vi "4Pi Objective Image Alignment.vi"(7 "Calling VI Ref":refnum<vi>) -> ()   [LabVIEW 2016]
uses:
  4Pi OIA - Controls/4Pi OIA - ROI Selection.ctl
  4Pi OIA - Controls/4Pi OIA - Method.ctl
  4Pi OIA - Controls/4Pi OIA - Default Settings.ctl
  <vilib>/vision/Image Controls.llb/IMAQ Image.ctl
  4Pi OIA - Controls/4Pi OIA - Notifier Type.ctl
  4Pi OIA - Controls/4Pi OIA - Actions.ctl
  <vilib>/Utility/miscctls.llb/LVPointTypeDef.ctl
  Hardware Configuration/Hardware Configuration Controls/Device Function.ctl
  Hardware Configuration/Hardware Configuration Controls/Device Type.ctl
  Device Library/Cameras/Hamamatsu/Orca Flash/Orca Flash Controls/Orca Flash Actions.ctl
  Device Library/Shutters/Shutter Controls/Shutter Actions.ctl
  Device Library/Stages/Stages Controls/Stage Actions.ctl
  <resource>/objmgr/IMAQImage.rc
panel:
  in  "Main Tab":enum32{"Objective Alignment", "Settings"}(tab)
  in  "ROI Selection":T1
  in  "Image Selection":i32(ring) items=["Quad 01", "Quad 02", "Quad 03", "Quad 04"]
  in  "Method":T2
  in  "Align":bool
  in  "Frame Accumulations":u16=10
  in  "Alignment Cycles":u16=1
  out "Move Limit Error":bool
  in  "Save Default Config":bool
  in  "Objective Flip Ctrl":T3={"Flip X and Y"=FALSE, "Invert X"=FALSE, "Invert Y"=FALSE, "Camera Px. Size (µm)"=0.1, "Objective Move Limit (µm)"=1.0}
  in  "Get Shift":bool
  in  "Quit":bool
  # "For Debuggin Only"
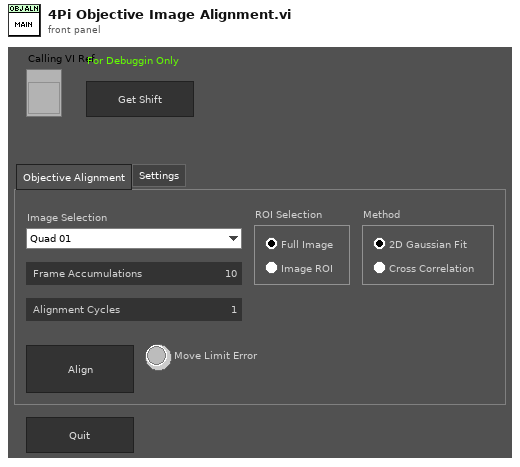
[diagram p1: front panel]
types:
  T1 = typedef "4Pi OIA - ROI Selection.ctl" = enum32{"Full Image", "ROI"}
  T2 = typedef "4Pi OIA - Method.ctl" = enum32{"2D Gaussian Fit", "Cross Correlation"}
  T3 = typedef "4Pi OIA - Default Settings.ctl" = cluster{"Flip X and Y":bool, "Invert X":bool, "Invert Y":bool, "Camera Px. Size (µm)":dbl, "Objective Move Limit (µm)":dbl}
  T4 = enum16{"Always On", "Always Off", "Off While Running"}
  T5 = typedef "LVPointTypeDef.ctl" = cluster{"Horizontal":i16, "Vertical":i16}
  T6 = typedef "4Pi OIA - Actions.ctl" = enum16{"Idle", "Start Alignment", "Get Upper Image", "Get Lower Image", "Get Shift", "Check Shift", "Move OBJ", "Quit"}
  T7 = enum8{"Enabled", "Disabled", "Disabled and Grayed Out"}
  T8 = typedef "4Pi OIA - Notifier Type.ctl" = cluster{"Action":T6, "ROI Selection":T1, "Method":T2, "Frame Accums.":u16, "Image Ref":T9, "OIA Default Settings":T3}
  T9 = typedef "IMAQ Image.ctl" = refnum<image>
  T10 = typedef "Device Function.ctl" = enum16{"Primary", "Secondary", "Overview", "Wide Field Drift Correction", "642 nm Excitation", "560 nm Excitation", "546 nm Excitation", "488 nm Excitation", "405 nm Excitation", "Objective Drift Correction", "Objective XY", "Objective Z", "Sample XY", "Sample Coarse Z", "Sample Z", "4Pi Lower", "4Pi Upper", "Adj Cavity", "Line Scanning", "Alert"}
  T11 = typedef "Device Type.ctl" = enum16{"AOTF", "Camera", "Deformable Mirror", "Laser", "Shutter", "Stage", "Waveform", "Email"}
  T12 = typedef "Orca Flash Actions.ctl" = enum16{"IDLE", "PREVIEW", "RECORD", "Record Settings", "SETPARAM", "GETPARAM", "SETROI", "GETROI", "PROGRESSIVE MODE", "AREA MODE", "STATUS", "QUIT"}
  T13 = typedef "Shutter Actions.ctl" = enum16{"Open", "Close", "Toggle", "Status", "Quit"}
  T14 = typedef "Stage Actions.ctl" = enum16{"Get Position", "MVR", "MOVE", "HALT", "ONTARGET", "ERROR", "REFERENCE", "INIT", "VELOCITY", "STATUS", "EXIT", "HOME", "ZEROPOS", "NANOPOS", "ANALOG", "QUIT"}
  T15 = enum32{"Invalid", "Standard", "Closed", "Hidden", "Minimized", "Maximized"}
  T16 = typedef "2D Gaussian - Best Fit Parameters.ctl" = cluster{"Amplitude":dbl, "X Position":dbl, "Y Position":dbl, "X Width":dbl, "Y Width":dbl, "Offset":dbl}
  T17 = typedef "LVRectTypeDef.ctl" = cluster{"Left":i16, "Top":i16, "Right":i16, "Bottom":i16}
  T18 = typedef "LVBoundsTypeDef.ctl" = cluster{"Width":u32, "Height":u32}
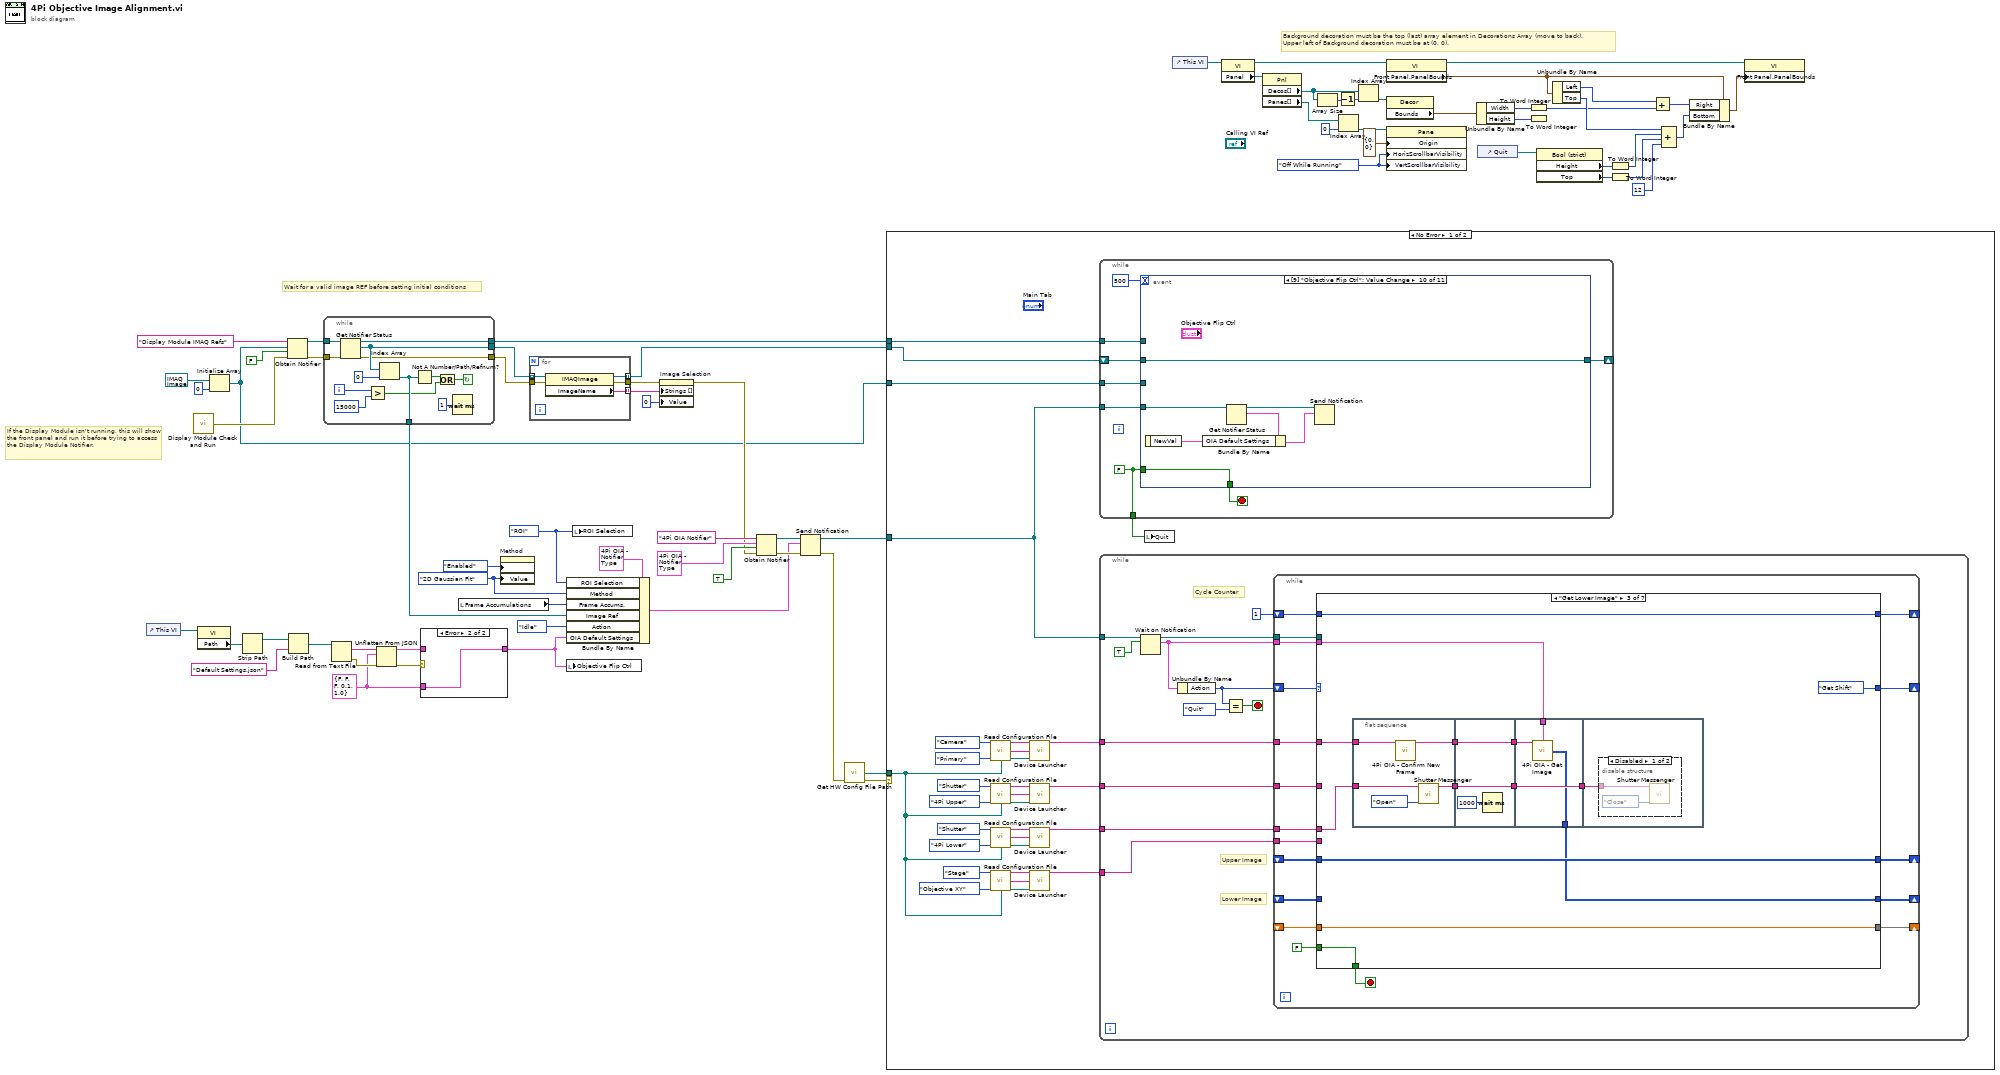
[diagram p0: block diagram]
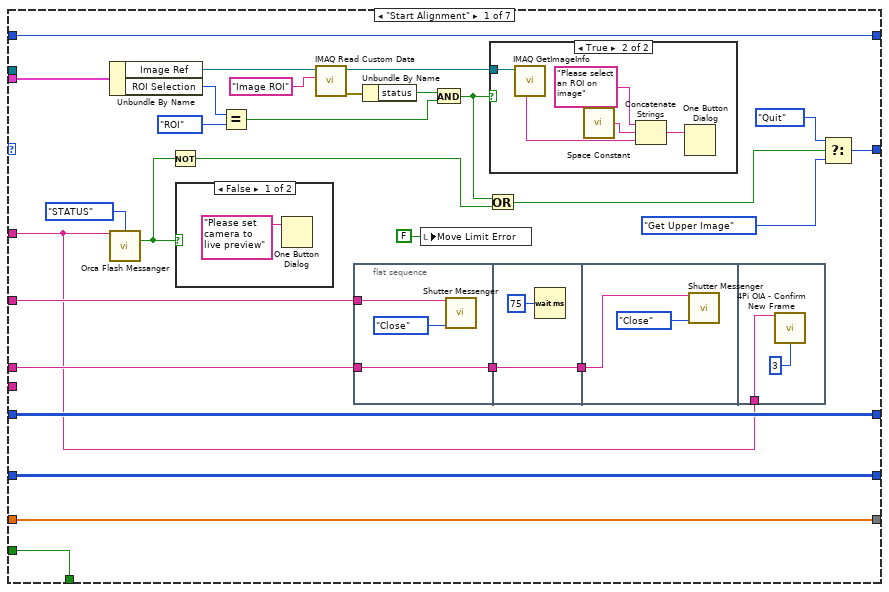
[diagram p3: hidden frame]
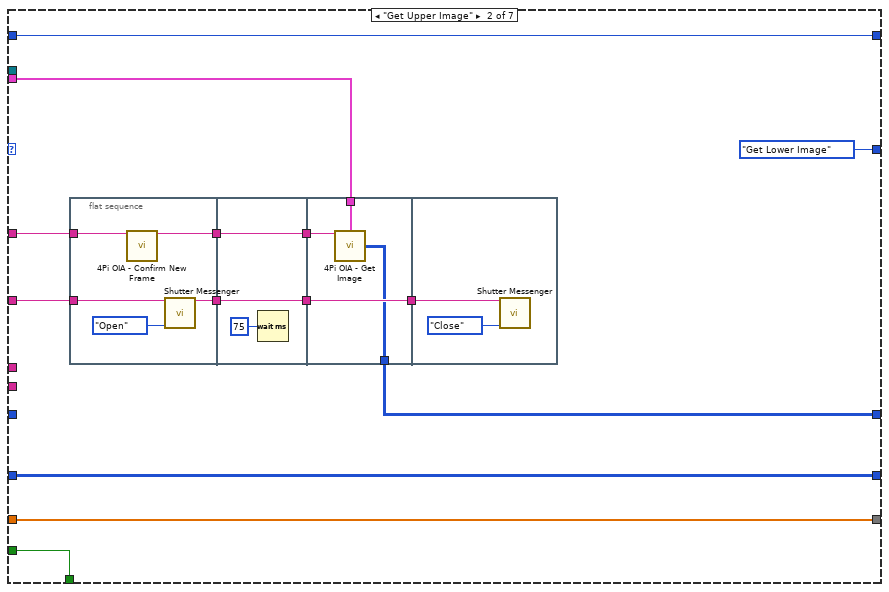
[diagram p6: hidden frame]
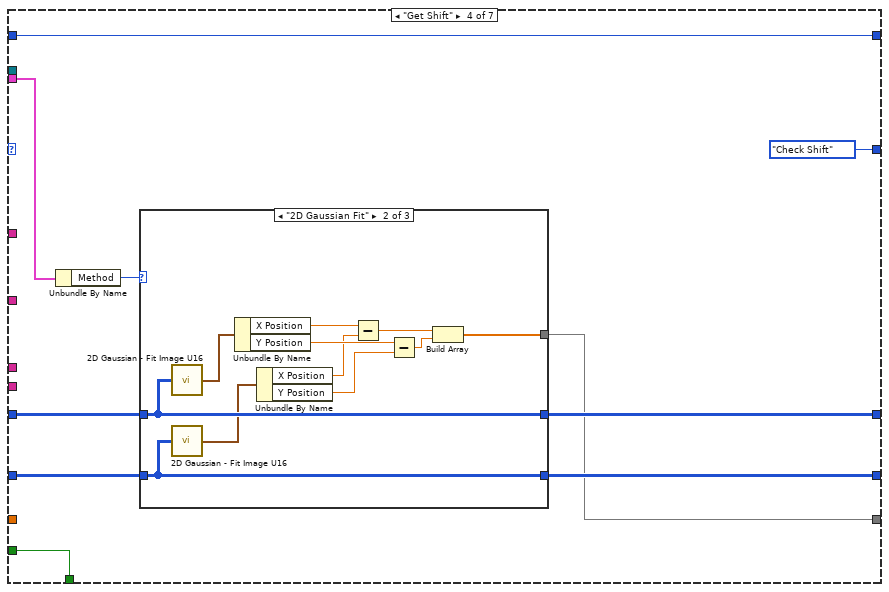
[diagram p8: hidden frame]
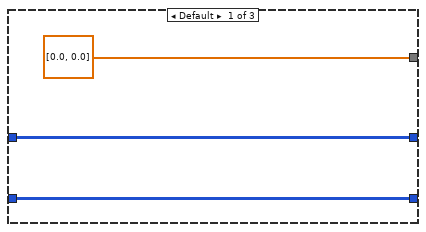
[diagram p9: hidden frame]
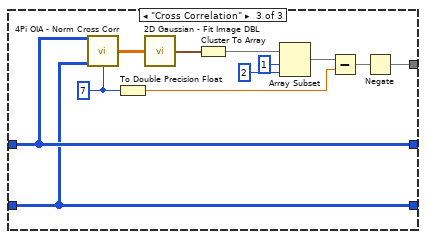
[diagram p10: hidden frame]
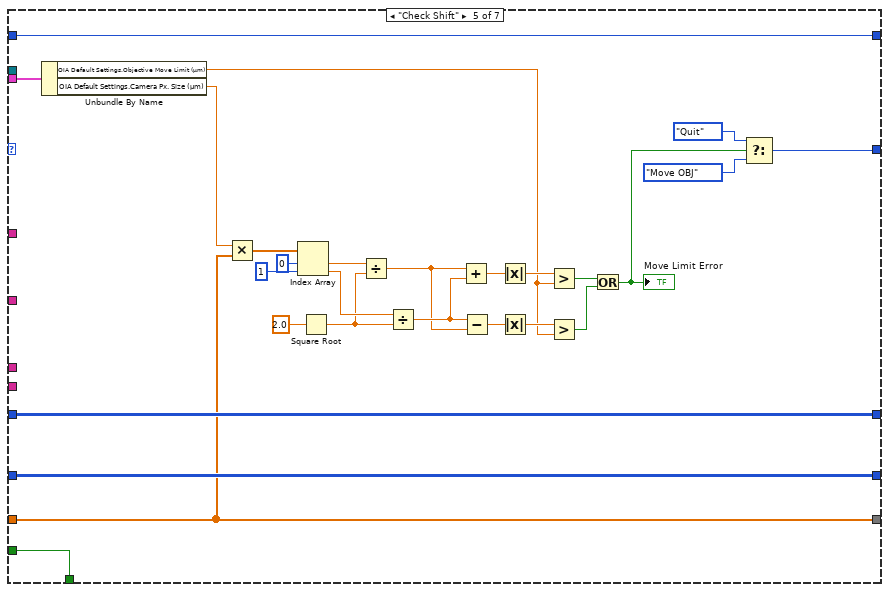
[diagram p11: hidden frame]
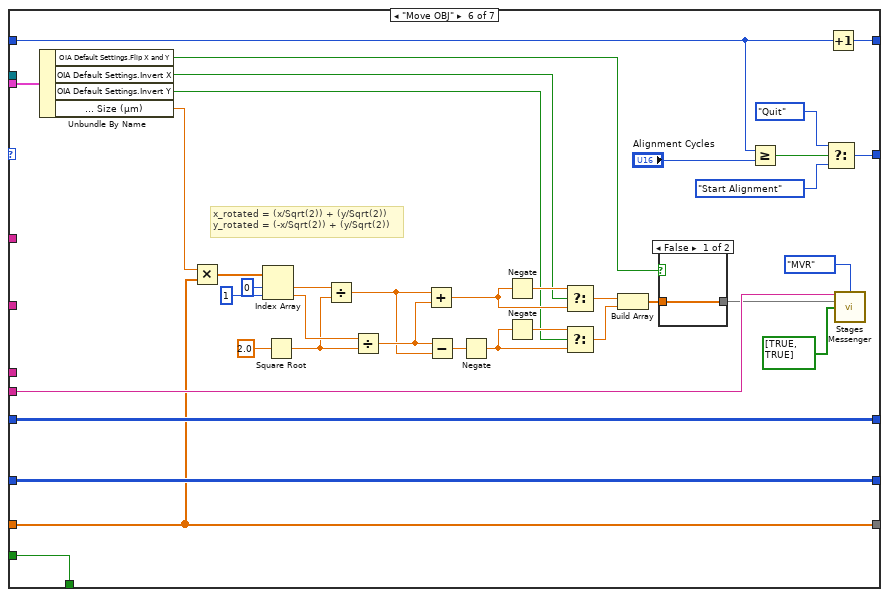
[diagram p12: hidden frame]
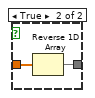
[diagram p13: hidden frame]
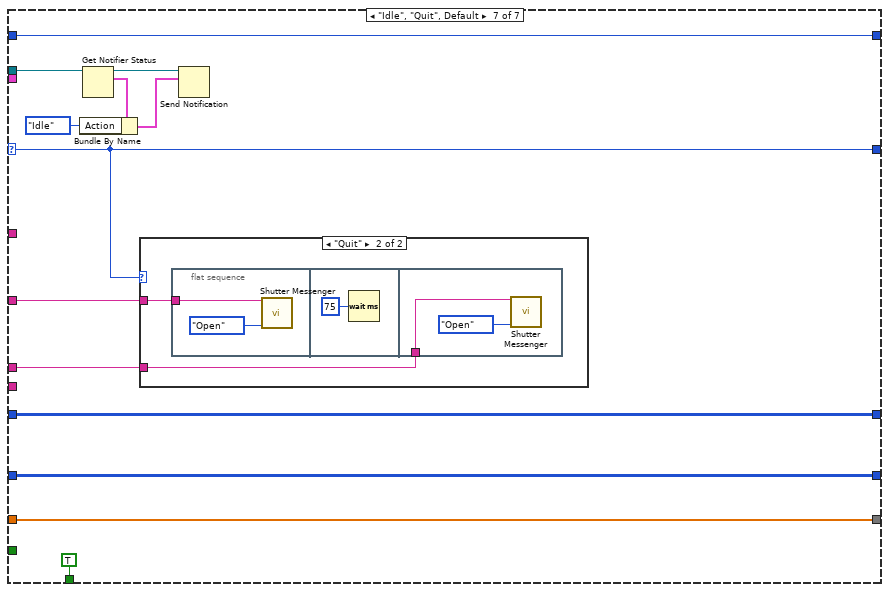
[diagram p14: hidden frame]
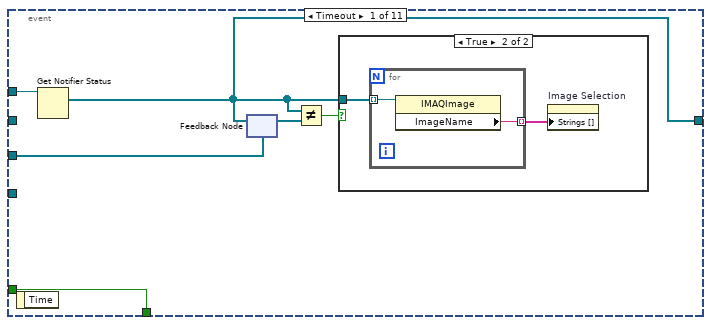
[diagram p16: hidden frame]
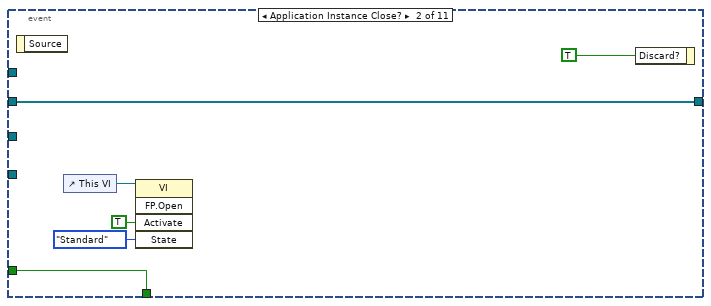
[diagram p18: hidden frame]
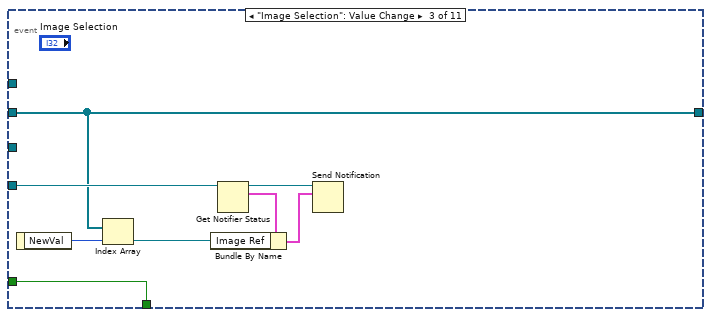
[diagram p19: hidden frame]
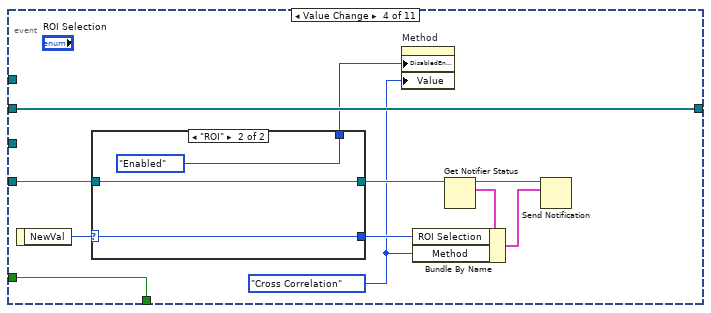
[diagram p20: hidden frame]
diagram:
  w2 = T3 {"Flip X and Y"=FALSE, "Invert X"=FALSE, "Invert Y"=FALSE, "Camera Px. Size (µm)"=0.1, "Objective Move Limit (µm)"=1.0} ("Objective Flip Type Def")
  w36 = T4."Off While Running" ("Vertical Scrollbar Visibility")
  w61 = 4Pi_OIA_-_Method."2D Gaussian Fit" ("Method")
  w62 = 4Pi_OIA_-_ROI_Selection."ROI" ("ROI Selection")
  # "Wait for a valid image REF before setting initial conditions"
  # "If the Display Module isn't running, this will show the front panel and run it before trying to access the Display Module Notifier."
  # "Background decoration must be the top (last) array element in Decorations Array (move to back).\nUpper left of Background decoration must be at (0, 0)."
  n1 = control-ref of="This VI"() -> (w8:refnum<vi>)
  n2 = call "Display Module Check and Run.vi"() -> ("Error"=w24:errorcluster)  [unwired: 15 in]
  n3 = property class="VI"(reference=w8) -> ("Path"=w9:path)  [unwired: 1 in, 2 out]
  n4 = Initialize Array(T9 refnum ("New Image"), 0 ("dimension size")) -> (w12:T9[])
  n5 = Strip Path(path=w9) -> (stripped path=w10:path)  [unwired: 1 out]
  n6 = Obtain Notifier(name (unnamed)="Display Module IMAQ Refs", notification data type=w12, create if not found? (T)=FALSE, error in (no error)=w24) -> (notifier out=w23:refnum<notifier>, error out=w22:errorcluster)  [unwired: 1 out]
  n7 = Build Path(base path=w10, name or relative path="Default Settings.json") -> (appended path=w7:path)
  n8 = while {
    tunnel: w23 -> [w86]
    tunnel: w22 -> [w85]
    tunnel: [w84] -> w21
    tunnel: [w83] -> w16
    tunnel: [w81] -> w20
    tunnel: [w79] -> w13
    i -> [w78]
    stop <- w75 continue-if-true
    n9 = Get Notifier Status(notifier=w86, error in (no error)=w85) -> (notifier out=w84:refnum<notifier>, current notification=w83:T9[], error out=w79:errorcluster)  [unwired: 2 out]
    n10 = Greater?(x=w78, y=15000) -> (0:w74:bool)
    n11 = Index Array(array=w83, index=0) -> (element=w81:T9)
    n12 = Not A Number/Path/Refnum?(number/path/refnum=w81) -> (NaN/Path/Refnum?=w76:bool)
    n13 = Or(x=w76, y=w74) -> (x .or. y?=w75:bool)
    n14 = Wait (ms)(milliseconds to wait=u32 1) -> ()  [unwired: 1 out]
  }
  n15 = Read from Text File(file (use dialog)=w7) -> (text=w6:string, error out=w5:errorcluster)  [unwired: 3 in, 2 out]
  n16 = Unflatten From JSON(JSON string=w6, type and defaults=w2, error in (no error)=w5) -> (value=w3:T3, error out=w4:errorcluster)  [unwired: 4 in]
  n17 = case shown="Error" w4 {
    tunnel: w3 -> [w87 _]
    tunnel: [w87 w88] -> w1
    tunnel: w2 -> [_ w88]
    frame No Error {
    }
    frame Error {
    }
  }
  n18 = local read "Frame Accumulations"() -> (w55:u16)
  n19 = property on="Method" class="RadioBtnsControl (strict)"("DisabledEnum"=T7."Enabled" ("Disabled"), "Value"=w61) -> ()  [unwired: 2 in, 2 out]
  n20 = for {
    tunnel: w16 -> [w93] mode=indexing
    tunnel: [w92] -> w19 mode=indexing
    tunnel: [w91] -> w17
    tunnel: [w90] -> w15 mode=indexing
    tunnel: w13 -> [w89]
    n21 = property class="IMAQImage"(reference=w93, error in=w89) -> (reference out=w90:T9, error out=w91:errorcluster, "ImageName"=w92:string)
  }
  n22 = Bundle By Name(cluster=T8 {"Action"=enum."Start Alignment", "ROI Selection"=enum."Full Image", "Method"=enum."2D Gaussian Fit", "Frame Accums."=0, "Image Ref"=refnum, "OIA Default Settings"={"Flip X and Y"=FALSE, "Invert X"=FALSE, "Invert Y"=FALSE, "Camera Px. Size (µm)"=0.1, "Objective Move Limit (µm)"=1.0}} ("4Pi OIA Notifier Type"), "ROI Selection"=w62, "Method"=w61, "Frame Accums."=w55, "Image Ref"=w20, "Action"=4Pi_OIA_-_Actions."Idle", "OIA Default Settings"=w1) -> (w57:T8)
  n23 = local write "Objective Flip Ctrl"(w1) -> ()
  n24 = local write "ROI Selection"(w62) -> ()
  n25 = property on="Image Selection" class="Ring (strict)"(error in=w17, "Strings []"=w19, "Value"=0) -> (error out=w14:errorcluster)  [unwired: 1 in, 1 out]
  n26 = Obtain Notifier(name (unnamed)="4Pi OIA Notifier", notification data type=T8 {"Action"=enum."Start Alignment", "ROI Selection"=enum."Full Image", "Method"=enum."2D Gaussian Fit", "Frame Accums."=0, "Image Ref"=refnum, "OIA Default Settings"={"Flip X and Y"=FALSE, "Invert X"=FALSE, "Invert Y"=FALSE, "Camera Px. Size (µm)"=0.1, "Objective Move Limit (µm)"=1.0}} ("4Pi OIA Notifier Type"), create if not found? (T)=TRUE, error in (no error)=w14) -> (notifier out=w60:refnum<notifier>, error out=w58:errorcluster)  [unwired: 1 out]
  n27 = Send Notification(notification=w57, notifier=w60, error in (no error)=w58) -> (notifier out=w59:refnum<notifier>, error out=w56:errorcluster)
  n28 = call "Get HW Config File Path.vi"("Error"=w56) -> ("File Path"=w72:path, "Error"=w73:errorcluster)  [unwired: 13 in]
  n29 = case shown="No Error" w73 {
    tunnel: w72 -> [w122 _]
    tunnel: w21 -> [w121 _]
    tunnel: w12 -> [w120 _]
    tunnel: w59 -> [w118 _]
    tunnel: w15 -> [w119 _]
    frame No Error {
      n30 = call "Read Configuration File.vi"("Device Type"=Device_Type."Camera", "Device Function"=Device_Function."Primary", "Config File Path"=w122) -> ("Unique Notifier Name"=w112:string, "Device Ports/IDs/Channels"=w114:string[], "Device Engine Path"=w113:path)  [unwired: 9 in, 1 out]
      n31 = call "Read Configuration File.vi"("Device Type"=Device_Type."Shutter", "Device Function"=Device_Function."4Pi Upper", "Config File Path"=w122) -> ("Unique Notifier Name"=w97:string, "Device Ports/IDs/Channels"=w99:string[], "Device Engine Path"=w98:path)  [unwired: 9 in, 1 out]
      n32 = call "Read Configuration File.vi"("Device Type"=Device_Type."Shutter", "Device Function"=Device_Function."4Pi Lower", "Config File Path"=w122) -> ("Unique Notifier Name"=w102:string, "Device Ports/IDs/Channels"=w100:string[], "Device Engine Path"=w101:path)  [unwired: 9 in, 1 out]
      n33 = call "Read Configuration File.vi"("Device Type"=Device_Type."Stage", "Device Function"=Device_Function."Objective XY", "Config File Path"=w122) -> ("Unique Notifier Name"=w107:string, "Device Ports/IDs/Channels"=w109:string[], "Device Engine Path"=w108:path)  [unwired: 9 in, 1 out]
      n34 = call "Device Launcher.vi"("Notifier Name"=w112, "Device Ports/IDs/Channels"=w114, "Device Engine Path"=w113) -> ("Notifier Name"=w117:string)  [unwired: 11 in, 1 out]
      n35 = call "Device Launcher.vi"("Notifier Name"=w97, "Device Ports/IDs/Channels"=w99, "Device Engine Path"=w98) -> ("Notifier Name"=w116:string)  [unwired: 11 in, 1 out]
      n36 = call "Device Launcher.vi"("Notifier Name"=w102, "Device Ports/IDs/Channels"=w100, "Device Engine Path"=w101) -> ("Notifier Name"=w115:string)  [unwired: 11 in, 1 out]
      n37 = call "Device Launcher.vi"("Notifier Name"=w107, "Device Ports/IDs/Channels"=w109, "Device Engine Path"=w108) -> ("Notifier Name"=w94:string)  [unwired: 11 in, 1 out]
      n38 = while {
        tunnel: [w382] -> w123
        tunnel: w121 -> [w381]
        tunnel: w120 -> [w380]
        tunnel: w118 -> [w379]
        shift-right: [w378] -> _
        shift-left: w119 -> [w377]
        stop <- w383 stop-if-true
        w382 = FALSE
        n39 = event shown="[9] \"Objective Flip Ctrl\": Value Change" {
          selector: _ -> [_ _ _ _ _ _ _ _ _ _ _]
          dyn-events: _ -> [_ _ _ _ _ _ _ _ _ _ _]
          timeout: 500 -> [_ _ _ _ _ _ _ _ _ _ _]
          tunnel: w382 -> [w390 w399 w408 w418 w432 w439 w446 w453 w463 w471 _]
          tunnel: [w390 w399 w408 w418 w432 w439 w446 w453 w463 w471 w478] -> w383
          tunnel: w381 -> [w389 _ _ _ _ _ _ _ _ _ _]
          tunnel: w380 -> [w388 _ _ _ _ _ _ _ _ _ _]
          tunnel: w379 -> [_ _ w407 w413 w427 w434 w445 w452 w462 w468 w472]
          tunnel: [w387 w395 w401 w419 w431 w438 w440 w447 w464 w469 w477] -> w378
          tunnel: w377 -> [_ w395 w401 w419 w431 w438 w440 w447 w464 w469 w477]
          event Timeout {
            n40 = event-data() -> ()  [unwired: 1 in, 1 out]
            n41 = Get Notifier Status(notifier=w389) -> (current notification=w387:T9[])  [unwired: 1 in, 4 out]
            n42 = feedback #1(w388) -> (w386:T9[])
            n43 = feedback-in #1(w387) -> ()
            n44 = Not Equal?(x=w387, y=w386) -> (x != y?=w385:bool)
            n45 = case shown="True" w385 {
              tunnel: w387 -> [_ w392]
              frame False {
              }
              frame True {
                n46 = for {
                  tunnel: w392 -> [w394] mode=indexing
                  tunnel: [w393] -> w391 mode=indexing
                  n47 = property class="IMAQImage"(reference=w394) -> ("ImageName"=w393:string)  [unwired: 1 in, 2 out]
                }
                n48 = property on="Image Selection" class="Ring (strict)"("Strings []"=w391) -> ()  [unwired: 2 in, 2 out]
              }
            }
          }
          event Application Instance Close? {
            n49 = event-data() -> ()  [unwired: 1 in, 1 out]
            n50 = control-ref of="This VI"() -> (w396:refnum<vi>)
            n51 = invoke class="VI" method="FP.Open"(reference=w396, "Activate"=TRUE ("Activate?"), "State"=T15."Standard") -> ()  [unwired: 2 in, 5 out]
            n52 = event-data("Discard?"=TRUE) -> ()  [unwired: 1 in, 1 out]
          }
          event "Image Selection": Value Change {
            n53 = event-data() -> ("NewVal"=w403:i32)  [unwired: 1 in]
            n54 = Index Array(array=w401, index=w403) -> (element=w402:T9)
            n55 = Get Notifier Status(notifier=w407) -> (notifier out=w406:refnum<notifier>, current notification=w405:T8)  [unwired: 1 in, 3 out]
            n56 = Bundle By Name(cluster=w405, "Image Ref"=w402) -> (w404:T8)
            n57 = Send Notification(notification=w404, notifier=w406) -> ()  [unwired: 1 in, 2 out]
          }
          event Value Change {
            w409 = 4Pi_OIA_-_Method."Cross Correlation" ("Method")
            n58 = event-data() -> ("NewVal"=w414:T1)  [unwired: 1 in]
            n59 = case shown="\"ROI\"" w414 {
              selector: w414 -> [w422 w424]
              tunnel: w413 -> [w421 w425]
              tunnel: [w422 w424] -> w411
              tunnel: [w421 w425] -> w412
              tunnel: [T7."Disabled and Grayed Out" ("Disabled") T7."Enabled" ("Disabled")] -> w410
              frame "Full Image", Default {
              }
              frame "ROI" {
              }
            }
            n60 = property on="Method" class="RadioBtnsControl (strict)"("DisabledEnum"=w410, "Value"=w409) -> ()  [unwired: 2 in, 2 out]
            n61 = Get Notifier Status(notifier=w412) -> (notifier out=w417:refnum<notifier>, current notification=w416:T8)  [unwired: 1 in, 3 out]
            n62 = Bundle By Name(cluster=w416, "ROI Selection"=w411, "Method"=w409) -> (w415:T8)
            n63 = Send Notification(notification=w415, notifier=w417) -> ()  [unwired: 1 in, 2 out]
          }
          event Value Change {
            n64 = event-data() -> ("NewVal"=w426:T2)  [unwired: 1 in]
            n65 = Get Notifier Status(notifier=w427) -> (notifier out=w430:refnum<notifier>, current notification=w429:T8)  [unwired: 1 in, 3 out]
            n66 = Bundle By Name(cluster=w429, "Method"=w426) -> (w428:T8)
            n67 = Send Notification(notification=w428, notifier=w430) -> ()  [unwired: 1 in, 2 out]
          }
          event "Frame Accumulations": Value Change {
            n68 = event-data() -> ("NewVal"=w433:u16)  [unwired: 1 in]
            n69 = Get Notifier Status(notifier=w434) -> (notifier out=w437:refnum<notifier>, current notification=w436:T8)  [unwired: 1 in, 3 out]
            n70 = Bundle By Name(cluster=w436, "Frame Accums."=w433) -> (w435:T8)
            n71 = Send Notification(notification=w435, notifier=w437) -> ()  [unwired: 1 in, 2 out]
          }
          event "Align": Value Change {
            n72 = event-data() -> ()  [unwired: 1 in, 1 out]
            n73 = Get Notifier Status(notifier=w445) -> (notifier out=w444:refnum<notifier>, current notification=w443:T8)  [unwired: 1 in, 3 out]
            n74 = Bundle By Name(cluster=w443, "Action"=4Pi_OIA_-_Actions."Start Alignment") -> (w442:T8)
            n75 = Send Notification(notification=w442, notifier=w444) -> ()  [unwired: 1 in, 2 out]
          }
          event "Get Shift": Value Change {
            # "For debugging only"
            n76 = event-data() -> ()  [unwired: 1 in, 1 out]
            n77 = Get Notifier Status(notifier=w452) -> (notifier out=w451:refnum<notifier>, current notification=w450:T8)  [unwired: 1 in, 3 out]
            n78 = Bundle By Name(cluster=w450, "Action"=4Pi_OIA_-_Actions."Get Shift") -> (w449:T8)
            n79 = Send Notification(notification=w449, notifier=w451) -> ()  [unwired: 1 in, 2 out]
          }
          event "Save Default Config": Value Change {
            n80 = event-data() -> ()  [unwired: 1 in, 1 out]
            n81 = Get Notifier Status(notifier=w462) -> (current notification=w456:T8)  [unwired: 1 in, 4 out]
            n82 = control-ref of="This VI"() -> (w461:refnum<vi>)
            n83 = Unbundle By Name(w456) -> ("OIA Default Settings"=w455:T3)
            n84 = property class="VI"(reference=w461) -> ("Path"=w460:path)  [unwired: 1 in, 2 out]
            n85 = Strip Path(path=w460) -> (stripped path=w459:path)  [unwired: 1 out]
            n86 = Flatten To JSON(anything=w455) -> (JSON string=w454:string)  [unwired: 2 in, 1 out]
            n87 = Build Path(base path=w459, name or relative path="Default Settings.json") -> (appended path=w457:path)
            n88 = Write to Text File(file (use dialog)=w457, text=w454) -> ()  [unwired: 2 in, 3 out]
          }
          event Value Change {
            n89 = event-data() -> ("NewVal"=w466:T3)  [unwired: 1 in]
            n90 = Get Notifier Status(notifier=w468) -> (notifier out=w470:refnum<notifier>, current notification=w467:T8)  [unwired: 1 in, 3 out]
            n91 = Bundle By Name(cluster=w467, "OIA Default Settings"=w466) -> (w465:T8)
            n92 = Send Notification(notification=w465, notifier=w470) -> ()  [unwired: 1 in, 2 out]
          }
          event "Quit": Value Change {
            n93 = event-data() -> ("NewVal"=w478:bool)  [unwired: 1 in]
            n94 = Get Notifier Status(notifier=w472) -> (notifier out=w473:refnum<notifier>, current notification=w474:T8)  [unwired: 1 in, 3 out]
            n95 = Bundle By Name(cluster=w474, "Action"=4Pi_OIA_-_Actions."Quit") -> (w475:T8)
            n96 = Send Notification(notification=w475, notifier=w473) -> ()  [unwired: 1 in, 2 out]
          }
        }
      }
      n97 = while {
        tunnel: w118 -> [w135]
        tunnel: w117 -> [w130]
        tunnel: w116 -> [w129]
        tunnel: w115 -> [w128]
        tunnel: w94 -> [w125]
        stop <- w132 stop-if-true
        # "Cycle Counter"
        # "Lower Image"
        # "Upper Image"
        n98 = Wait on Notification(notifier=w135, ignore previous (F)=TRUE) -> (notifier out=w126:refnum<notifier>, notification=w127:T8)  [unwired: 2 in, 2 out]
        n99 = Unbundle By Name(w127) -> ("Action"=w131:T6)
        n100 = Equal?(x=w131, y=4Pi_OIA_-_Actions."Quit") -> (x = y?=w132:bool)
        n101 = while {
          shift-right: [w150] -> _
          shift-left: w131 -> [w153]
          tunnel: w130 -> [w149]
          tunnel: w129 -> [w148]
          tunnel: w128 -> [w147]
          shift-right: [w144] -> _
          shift-left: _ -> [w143]
          shift-right: [w146] -> _
          shift-left: _ -> [w145]
          tunnel: w127 -> [w142]
          tunnel: w126 -> [w141]
          tunnel: w125 -> [w140]
          shift-right: [w139] -> _
          shift-left: _ -> [w138]
          shift-right: [w136] -> _
          shift-left: u16 1 -> [w137]
          stop <- w151 stop-if-true
          n102 = case shown="\"Get Lower Image\"" w153 {
            selector: w153 -> [_ _ _ _ _ _ w359]
            tunnel: FALSE -> [w181 w209 w237 w262 w315 w353 _]
            tunnel: [w181 w209 w237 w262 w315 w353 TRUE] -> w151
            tunnel: [w166 4Pi_OIA_-_Actions."Get Lower Image" ("Action") 4Pi_OIA_-_Actions."Get Shift" ("Action") 4Pi_OIA_-_Actions."Check Shift" ("Action") w291 w332 w359] -> w150
            tunnel: w149 -> [w158 w200 w231 _ _ _ _]
            tunnel: w148 -> [w164 w208 _ _ _ _ w358]
            tunnel: w147 -> [w163 _ w228 _ _ _ w357]
            tunnel: [w160 w202 w229 w256 w313 w351 w367] -> w146
            tunnel: w145 -> [w160 w202 _ w258 w313 w351 w367]
            tunnel: [w159 w201 w230 w257 w314 w352 w368] -> w144
            tunnel: w143 -> [w159 _ w230 w259 w314 w352 w368]
            tunnel: w142 -> [w157 w199 w227 w260 w302 w329 _]
            tunnel: w141 -> [_ _ _ _ _ _ w362]
            tunnel: w140 -> [_ _ _ _ _ w350 _]
            tunnel: [w156 w198 w226 w255 w303 w338 w361] -> w139
            tunnel: w138 -> [w156 w198 w226 _ w303 w338 w361]
            tunnel: w137 -> [w155 w197 w225 w254 w316 w331 w360]
            tunnel: [w155 w197 w225 w254 w316 w330 w360] -> w136
            frame "Start Alignment" {
              n103 = Unbundle By Name(w157) -> ("Image Ref"=w178:T9, "ROI Selection"=w180:T1)
              n104 = call "Orca Flash Messanger.vi"("Notifier Name"=w158, "Camera Actions"=Orca_Flash_Actions."STATUS") -> ("Running?"=w170:bool)  [unwired: 9 in, 4 out]
              n105 = Not(x=w170) -> (.not. x?=w169:bool)
              n106 = case shown="False" w170 {
                frame False {
                  n107 = One Button Dialog(message="Please set camera to live preview") -> ()  [unwired: 1 in, 1 out]
                }
                frame True {
                }
              }
              n108 = Equal?(x=w180, y=4Pi_OIA_-_ROI_Selection."ROI") -> (x = y?=w174:bool)
              n109 = call "IMAQ Read Custom Data"("Key"="Image ROI", "Image"=w178) -> ("error out"=w176:errorcluster, "Image (duplicate)"=w173:T9)  [unwired: 7 in, 1 out]
              n110 = flat-sequence {
                tunnel: w164 -> [w183]
                tunnel: w163 -> [w182]
                tunnel: [w182] -> w162
                tunnel: w162 -> [w186]
                tunnel: [w186] -> w161
                tunnel: w161 -> [w187]
                tunnel: w158 -> [w190]
                frame #0 {
                  n111 = call "Shutter Messenger.vi"("Notifier Name"=w183, "Action"=Shutter_Actions."Close") -> ()  [unwired: 12 in, 2 out]
                }
                frame #1 {
                  n112 = Wait (ms)(milliseconds to wait=u32 75) -> ()  [unwired: 1 out]
                }
                frame #2 {
                  n113 = call "Shutter Messenger.vi"("Notifier Name"=w187, "Action"=Shutter_Actions."Close") -> ()  [unwired: 12 in, 2 out]
                }
                frame #3 {
                  n114 = call "4Pi OIA - Confirm New Frame.vi"("Camera Notifier Name"=w190, "Wait No. (1)"=u32 3 ("Wait No.")) -> ()  [unwired: 13 in, 1 out]
                }
              }
              n115 = Unbundle By Name(w176) -> ("status"=w175:bool)
              n116 = local write "Move Limit Error"(FALSE ("Move Limit Error")) -> ()
              n117 = And(x=w175, y=w174) -> (x .and. y?=w171:bool)
              n118 = Or(x=w171, y=w169) -> (x .or. y?=w168:bool)
              n119 = case shown="True" w171 {
                tunnel: w173 -> [_ w196]
                frame False {
                }
                frame True {
                  n120 = call "IMAQ GetImageInfo"("Image"=w196) -> ("Image Name"=w195:string)  [unwired: 3 in, 7 out]
                  n121 = call <vilib>:"Space Constant.vi"() -> ("String"=w194:string)
                  n122 = Concatenate Strings("Please select an ROI on image", w194, w195) -> (w192:string)
                  n123 = One Button Dialog(message=w192) -> ()  [unwired: 1 in, 1 out]
                }
              }
              n124 = Select(t=4Pi_OIA_-_Actions."Quit" ("Action"), s=w168, f=4Pi_OIA_-_Actions."Get Upper Image") -> (s? t:f=w166:T6)
            }
            frame "Get Upper Image" {
              n125 = flat-sequence {
                tunnel: [w213] -> w205
                tunnel: [w211] -> w203
                tunnel: w208 -> [w214]
                tunnel: w200 -> [w212]
                tunnel: [w218] -> w206
                tunnel: w205 -> [w218]
                tunnel: [w216] -> w204
                tunnel: w203 -> [w216]
                tunnel: [w222] -> w207
                tunnel: w206 -> [w222]
                tunnel: w204 -> [w221]
                tunnel: w199 -> [w220]
                tunnel: [w219] -> w201
                tunnel: w207 -> [w223]
                frame #0 {
                  n126 = call "4Pi OIA - Confirm New Frame.vi"("Camera Notifier Name"=w212) -> ("Camera Notifier Name (Dup)"=w211:string)  [unwired: 14 in]
                  n127 = call "Shutter Messenger.vi"("Notifier Name"=w214, "Action"=Shutter_Actions."Open") -> ("Notifier Name Dup"=w213:string)  [unwired: 12 in, 1 out]
                }
                frame #1 {
                  n128 = Wait (ms)(milliseconds to wait=u32 75) -> ()  [unwired: 1 out]
                }
                frame #2 {
                  n129 = call "4Pi OIA - Get Image.vi"("Camera Notifier Name"=w221, "Alignment Data"=w220) -> ("Image Out"=w219:u16[][])  [unwired: 13 in]
                }
                frame #3 {
                  n130 = call "Shutter Messenger.vi"("Notifier Name"=w223, "Action"=Shutter_Actions."Close") -> ()  [unwired: 12 in, 2 out]
                }
              }
            }
            frame "Get Lower Image" {
              n131 = flat-sequence {
                tunnel: [w242] -> w234
                tunnel: [w239] -> w232
                tunnel: w231 -> [w240]
                tunnel: w228 -> [w241]
                tunnel: [w246] -> w235
                tunnel: w234 -> [w246]
                tunnel: [w244] -> w233
                tunnel: w232 -> [w244]
                tunnel: [w250] -> w236
                tunnel: w235 -> [w250]
                tunnel: w233 -> [w249]
                tunnel: w227 -> [w248]
                tunnel: [w247] -> w229
                tunnel: w236 -> [w251]
                frame #0 {
                  n132 = call "4Pi OIA - Confirm New Frame.vi"("Camera Notifier Name"=w240) -> ("Camera Notifier Name (Dup)"=w239:string)  [unwired: 14 in]
                  n133 = call "Shutter Messenger.vi"("Notifier Name"=w241, "Action"=Shutter_Actions."Open") -> ("Notifier Name Dup"=w242:string)  [unwired: 12 in, 1 out]
                }
                frame #1 {
                  n134 = Wait (ms)(milliseconds to wait=u32 1000) -> ()  [unwired: 1 out]
                }
                frame #2 {
                  n135 = call "4Pi OIA - Get Image.vi"("Camera Notifier Name"=w249, "Alignment Data"=w248) -> ("Image Out"=w247:u16[][])  [unwired: 13 in]
                }
                frame #3 {
                  n136 = disable-structure shown="Disabled" {
                    disable-tunnel: w251 -> [w252 _]
                    frame Disabled {
                      n137 = call "Shutter Messenger.vi"("Notifier Name"=w252, "Action"=Shutter_Actions."Close") -> ()  [unwired: 12 in, 2 out]
                    }
                    frame Enabled {
                    }
                  }
                }
              }
            }
            frame "Get Shift" {
              n138 = Unbundle By Name(w260) -> ("Method"=w261:T2)
              n139 = case shown="\"2D Gaussian Fit\"" w261 {
                tunnel: w259 -> [w266 w277 w289]
                tunnel: w258 -> [w265 w276 w288]
                tunnel: [w266 w277 w289] -> w257
                tunnel: [w265 w276 w288] -> w256
                tunnel: [dbl[] [0.0, 0.0] w268 w278] -> w255
                frame Default {
                }
                frame "2D Gaussian Fit" {
                  n140 = call "2D Gaussian - Fit Image U16.vi"("Image In (U16)"=w277) -> ("Best Fit Params"=w267:T16)  [unwired: 13 in, 1 out]
                  n141 = call "2D Gaussian - Fit Image U16.vi"("Image In (U16)"=w276) -> ("Best Fit Params"=w275:T16)  [unwired: 13 in, 1 out]
                  n142 = Unbundle By Name(w267) -> ("X Position"=w274:dbl, "Y Position"=w273:dbl)
                  n143 = Unbundle By Name(w275) -> ("X Position"=w272:dbl, "Y Position"=w271:dbl)
                  n144 = Subtract(x=w274, y=w272) -> (x-y=w270:dbl)
                  n145 = Subtract(x=w273, y=w271) -> (x-y=w269:dbl)
                  n146 = Build Array(w270, w269) -> (w268:dbl[])
                }
                frame "Cross Correlation" {
                  w282 = 7 ("Half Shift")
                  n147 = call "4Pi OIA - Norm Cross Corr.vi"("Image 01"=w289, "Image 02"=w288, "Half Shift"=w282) -> ("Norm Cross Corr Result"=w287:dbl[][])  [unwired: 12 in]
                  n148 = To Double Precision Float(number=w282) -> (double precision float=w280:dbl)
                  n149 = call "2D Gaussian - Fit Image DBL.vi"("Image In (DBL)"=w287) -> ("Best Fit Params"=w286:T16)  [unwired: 13 in, 1 out]
                  n150 = Cluster To Array(cluster=w286) -> (array=w285:dbl[])
                  n151 = Array Subset(array=w285, index=1, length=2) -> (w281:dbl[])
                  n152 = Subtract(x=w281, y=w280) -> (x-y=w279:dbl[])
                  n153 = Negate(x=w279) -> (-x=w278:dbl[])
                }
              }
            }
            frame "Check Shift" {
              n154 = Unbundle By Name(w302) -> ("OIA Default Settings.Objective Move Limit (µm)"=w296:dbl, "OIA Default Settings.Camera Px. Size (µm)"=w301:dbl)
              n155 = Multiply(x=w301, y=w303) -> (x*y=w304:dbl[])
              n156 = Index Array(array=w304, index #1=0 ("index"), index #2=1 ("index")) -> (element #1=w310:dbl, element #2=w308:dbl)
              n157 = Square Root(x=2.0) -> (sqrt(x)=w307:dbl)
              n158 = Divide(x=w310, y=w307) -> (x/y=w305:dbl)
              n159 = Divide(x=w308, y=w307) -> (x/y=w306:dbl)
              n160 = Add(x=w305, y=w306) -> (x+y=w300:dbl)
              n161 = Subtract(x=w306, y=w305) -> (x-y=w299:dbl)
              n162 = Absolute Value(x=w300) -> (abs(x)=w298:dbl)
              n163 = Absolute Value(x=w299) -> (abs(x)=w297:dbl)
              n164 = Greater?(x=w298, y=w296) -> (0:w295:bool)
              n165 = Greater?(x=w297, y=w296) -> (0:w294:bool)
              n166 = Or(x=w295, y=w294) -> (x .or. y?=w290:bool)
              "Move Limit Error" <- w290
              n167 = Select(t=4Pi_OIA_-_Actions."Quit" ("Action"), s=w290, f=4Pi_OIA_-_Actions."Move OBJ" ("Action")) -> (s? t:f=w291:T6)
            }
            frame "Move OBJ" {
              # "x_rotated = (x/Sqrt(2)) + (y/Sqrt(2))\ny_rotated = (-x/Sqrt(2)) + (y/Sqrt(2))"
              n168 = Unbundle By Name(w329) -> ("OIA Default Settings.Flip X and Y"=w326:bool, "OIA Default Settings.Invert X"=w318:bool, "OIA Default Settings.Invert Y"=w319:bool, "OIA Default Settings.Camera Px. Size (µm)"=w336:dbl)
              n169 = Multiply(x=w336, y=w338) -> (x*y=w337:dbl[])
              n170 = Index Array(array=w337, index #1=0 ("index"), index #2=1 ("index")) -> (element #1=w345:dbl, element #2=w343:dbl)
              n171 = Square Root(x=2.0) -> (sqrt(x)=w342:dbl)
              n172 = Divide(x=w345, y=w342) -> (x/y=w340:dbl)
              n173 = Divide(x=w343, y=w342) -> (x/y=w341:dbl)
              n174 = Add(x=w340, y=w341) -> (x+y=w323:dbl)
              n175 = Subtract(x=w341, y=w340) -> (x-y=w339:dbl)
              n176 = Negate(x=w339) -> (-x=w320:dbl)
              n177 = Negate(x=w323) -> (-x=w322:dbl)
              n178 = Negate(x=w320) -> (-x=w321:dbl)
              n179 = Select(t=w322, s=w318, f=w323) -> (s? t:f=w325:dbl)
              n180 = Select(t=w321, s=w319, f=w320) -> (s? t:f=w324:dbl)
              n181 = Build Array(w325, w324) -> (w328:dbl[])
              n182 = case shown="False" w326 {
                tunnel: w328 -> [w354 w356]
                tunnel: [w354 w355] -> w327
                frame False {
                }
                frame True {
                  n183 = Reverse 1D Array(array=w356) -> (reversed array=w355:dbl[])
                }
              }
              n184 = Greater Or Equal?(x=w331, y="Alignment Cycles") -> (x >= y?=w333:bool)
              n185 = Select(t=4Pi_OIA_-_Actions."Quit" ("Action"), s=w333, f=4Pi_OIA_-_Actions."Start Alignment" ("Action")) -> (s? t:f=w332:T6)
              n186 = Increment(x=w331) -> (x+1=w330:u16)
              n187 = call "Stages Messenger.vi"("Stage Notifier Name"=w350, "Actions"=Stage_Actions."MVR", "Setpoint"=w327, "Axis"=bool[] [TRUE, TRUE]) -> ()  [unwired: 8 in, 4 out]
            }
            frame "Idle", "Quit", Default {
              n188 = Get Notifier Status(notifier=w362) -> (notifier out=w366:refnum<notifier>, current notification=w365:T8)  [unwired: 1 in, 3 out]
              n189 = Bundle By Name(cluster=w365, "Action"=4Pi_OIA_-_Actions."Idle") -> (w364:T8)
              n190 = case shown="\"Quit\"" w359 {
                tunnel: w358 -> [_ w371]
                tunnel: w357 -> [_ w370]
                frame Default {
                }
                frame "Quit" {
                  n191 = flat-sequence {
                    tunnel: w371 -> [w372]
                    tunnel: w370 -> [w375]
                    frame #0 {
                      n192 = call "Shutter Messenger.vi"("Notifier Name"=w372, "Action"=Shutter_Actions."Open") -> ()  [unwired: 12 in, 2 out]
                    }
                    frame #1 {
                      n193 = Wait (ms)(milliseconds to wait=u32 75) -> ()  [unwired: 1 out]
                    }
                    frame #2 {
                      n194 = call "Shutter Messenger.vi"("Notifier Name"=w375, "Action"=Shutter_Actions."Open") -> ()  [unwired: 12 in, 2 out]
                    }
                  }
                }
              }
              n195 = Send Notification(notification=w364, notifier=w366) -> ()  [unwired: 1 in, 2 out]
            }
          }
        }
      }
      n196 = local write "Quit"(w123) -> ()
    }
    frame Error {
      n197 = One Button Dialog(message="Objective image alignment tool failed to start.") -> ()  [unwired: 1 in, 1 out]
    }
  }
  n198 = control-ref of="This VI"() -> (w28:refnum<vi>)
  n199 = property class="VI"(reference=w28) -> (reference out=w37:refnum<vi>, "Panel"=w29:refnum<vi>)  [unwired: 1 in, 1 out]
  n200 = property class="Pnl"(reference=w29) -> ("Decos[]"=w27:refnum<vi>[], "Panes[]"=w33:refnum<vi>[])  [unwired: 1 in, 2 out]
  n201 = Array Size(array=w27) -> (size(s)=w25:i32)
  n202 = Decrement(x=w25) -> (x-1=w26:i32)
  n203 = Index Array(array=w33, index=0) -> (element=w32:refnum<vi>)
  n204 = Index Array(array=w27, index=w26) -> (element=w35:refnum<vi>)
  n205 = property class="VI"(reference=w37) -> (reference out=w39:refnum<vi>, "Front Panel.PanelBounds"=w40:T17)  [unwired: 1 in, 1 out]
  n206 = property class="Decor"(reference=w35) -> ("Bounds"=w38:T18)  [unwired: 1 in, 2 out]
  n207 = property class="Pane"(reference=w32, "Origin"=T5 {"Horizontal"=0, "Vertical"=0}, "HorizScrollbarVisibility"=w36, "VertScrollbarVisibility"=w36) -> ()  [unwired: 1 in, 2 out]
  n208 = Unbundle By Name(w38) -> ("Width"=w43:u32, "Height"=w46:u32)
  n209 = control-ref of="Quit"() -> (w30:refnum<vi>)
  n210 = To Word Integer(number=w43) -> (16bit integer=w45:i16)
  n211 = To Word Integer(number=w46) -> ()  [unwired: 1 out]
  n212 = property class="Bool (strict)"(reference=w30) -> ("Height"=w48:u32, "Top"=w49:i32)  [unwired: 1 in, 2 out]
  n213 = Unbundle By Name(w40) -> ("Left"=w42:i16, "Top"=w53:i16)
  n214 = To Word Integer(number=w48) -> (16bit integer=w51:i16)
  n215 = To Word Integer(number=w49) -> (16bit integer=w52:i16)
  n216 = Add(x=w42, y=w45) -> (x+y=w44:i16)
  n217 = Compound Arithmetic op=ADD(w53, w51, w52, i16 12 ("y")) -> (w47:i16)
  n218 = Bundle By Name(cluster=w40, "Right"=w44, "Bottom"=w47) -> (w41:T17)
  n219 = property class="VI"(reference=w39, "Front Panel.PanelBounds"=w41) -> ()  [unwired: 1 in, 2 out]
